vi "thcd_chan_all.vi"(8 "err_in":errorcluster, 9 "thcd_b2r":u32, 10 "thcd_delay":u32=500, 11 "thcd_visa":refnum<visa-resource-name>) -> (3 "thcd_res_1":T2, 4 "thcd_st":bool, 5 "thcd_res_str":string, 6 "err_out":errorcluster, 7 "thcd_visa":refnum<visa-resource-name>)   [LabVIEW 2020, in "1039_mod.lvlib"]
uses:
  1039_mod/1039_mod.lvlib
  thcd_controls/ctrl_chn_thcd.ctl
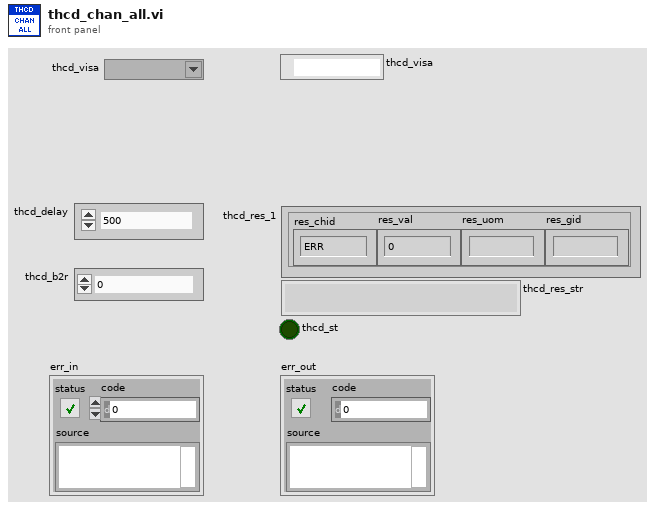
[diagram p1: front panel]
types:
  T1 = typedef "ctrl_chn_thcd.ctl" = enum8{"ERR", "1", "2", "3", "4"}
  T2 = cluster{"res_chid":T1, "res_val":dbl, "res_uom":string, "res_gid":string}
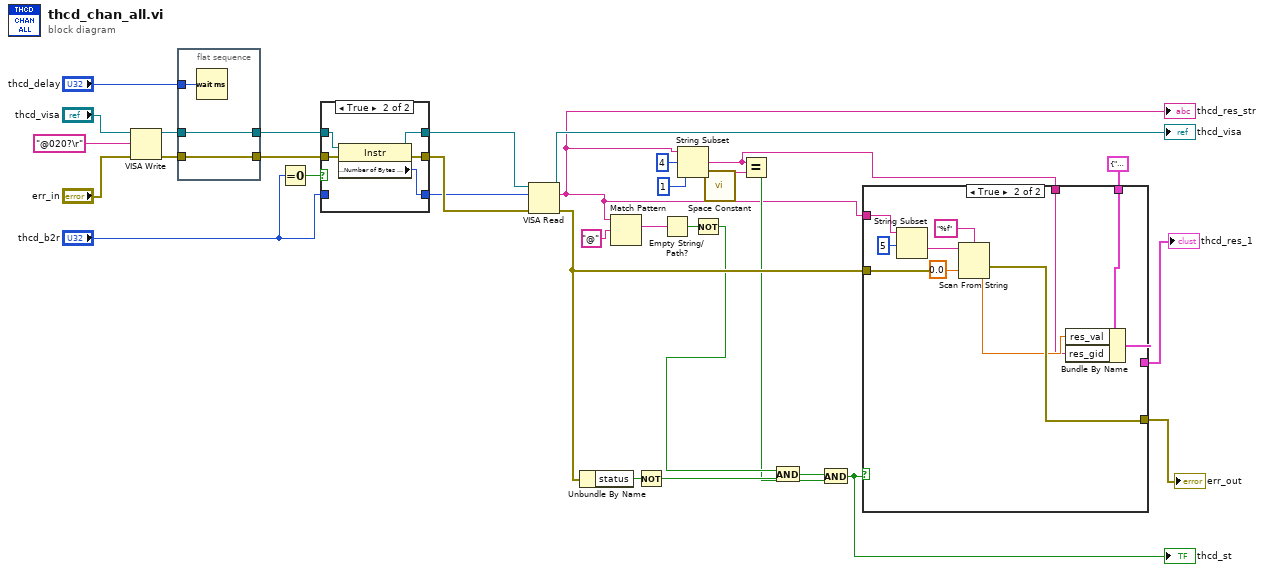
[diagram p0: block diagram]
diagram:
  n1 = VISA Write(VISA resource name="thcd_visa", write buffer="@020?\r" ("format string"), error in (no error)="err_in") -> (VISA resource name out=w31:refnum<visa-resource-name>, error out=w32:errorcluster)  [unwired: 1 out]
  n2 = flat-sequence {
    tunnel: w32 -> [w34]
    tunnel: [w34] -> w25
    tunnel: w31 -> [w33]
    tunnel: [w33] -> w26
    tunnel: "thcd_delay" -> [w35]
    frame #0 {
      n3 = Wait (ms)(milliseconds to wait=w35) -> ()  [unwired: 1 out]
    }
  }
  n4 = Equal To 0?(x="thcd_b2r") -> (x = 0?=w27:bool)
  n5 = case shown="True" w27 {
    tunnel: [w37 w43] -> w24
    tunnel: [w36 w42] -> w23
    tunnel: [w38 w41] -> w22
    tunnel: "thcd_b2r" -> [w38 _]
    tunnel: w26 -> [w37 w40]
    tunnel: w25 -> [w36 w39]
    frame False {
    }
    frame True {
      n6 = property class="Instr"(reference=w40, error in=w39) -> (reference out=w43:refnum<visa-resource-name>, error out=w42:errorcluster, "Serial Settings:Number of Bytes at Serial Port"=w41:u32)
    }
  }
  n7 = VISA Read(VISA resource name=w24, byte count=w22, error in (no error)=w23) -> (VISA resource name out=→"thcd_visa":refnum<visa-resource-name>, read buffer=w2:string, error out=w14:errorcluster)  [unwired: 1 out]
  "thcd_res_str" <- w2
  n8 = Unbundle By Name(w14) -> ("status"=w17:bool)
  n9 = Match Pattern(string=w2, regular expression="@") -> (match substring=w11:string)  [unwired: 1 in, 3 out]
  n10 = Not(x=w17) -> (.not. x?=w16:bool)
  n11 = Empty String/Path?(string/path=w11) -> (empty?=w10:bool)
  n12 = String Subset(string=w2, offset (0)=4, length (rest)=1 ("length (rest)")) -> (substring=w1:string)
  n13 = Not(x=w10) -> (.not. x?=w6:bool)
  n14 = call <vilib>:"Space Constant.vi"() -> ("String"=w7:string)
  n15 = Equal?(x=w1, y=w7) -> (x = y?=w5:bool)
  n16 = And(x=w6, y=w16) -> (x .and. y?=w4:bool)
  n17 = And(x=w4, y=w5) -> (x .and. y?=w3:bool)
  "thcd_st" <- w3
  n18 = case shown="True" w3 {
    tunnel: w2 -> [_ w48]
    tunnel: [w45 w53] -> w13
    tunnel: T2 {"res_chid"=enum."ERR", "res_val"=0.0, "res_uom"="", "res_gid"=""} ("res_1 2") -> [w45 w56]
    tunnel: w14 -> [w44 w49]
    tunnel: [w44 w52] -> w18
    tunnel: w1 -> [_ w46]
    frame False {
    }
    frame True {
      n19 = String Subset(string=w48, offset (0)=5) -> (substring=w50:string)  [unwired: 1 in]
      n20 = Scan From String(format string="%f", input string=w50, error in=w49, default 1=0.0 ("default value 1")) -> (error out=w52:errorcluster, output 1=w47:dbl)  [unwired: 1 in, 2 out]
      n21 = Bundle By Name(cluster=w56, "res_val"=w47, "res_gid"=w46) -> (w53:T2)
    }
  }
  "err_out" <- w18
  "thcd_res_1" <- w13
